vi "FWHM.vi"(3 "Peak Location":dbl, 4 "Intensity Data":dbl[](array[numeric])) -> (0 "Half Width XY Plot":cluster{dbl[], dbl[]}, 1 "Width":dbl)   [LabVIEW 2012]
panel:
  out "50% Mag - left index":dbl
  out "50% Mag - right index":dbl
  out "center -> left":dbl[](graph)
  out "center -> right":dbl[](graph)
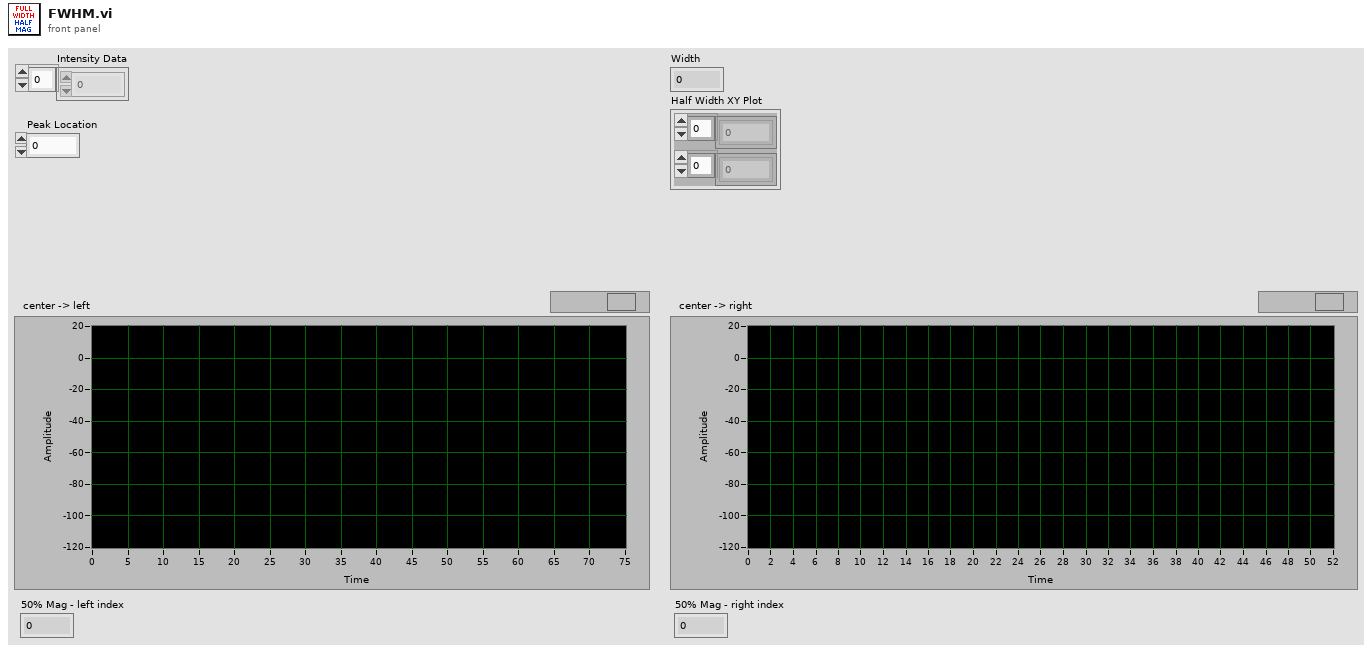
[diagram p1: front panel]
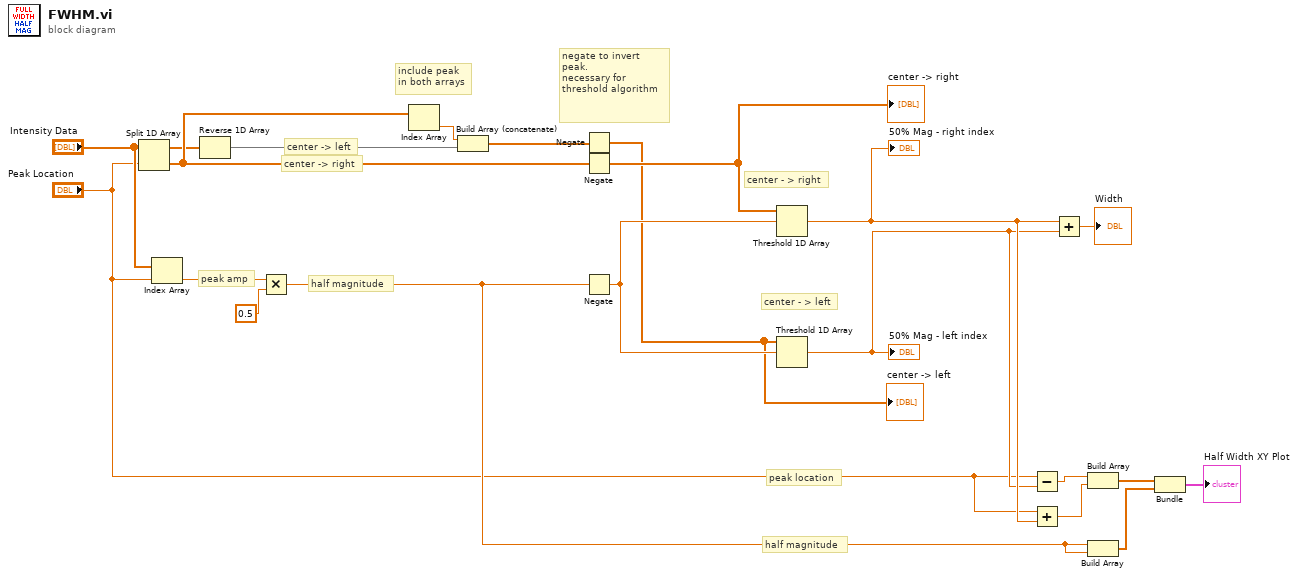
[diagram p0: block diagram]
diagram:
  # "peak amp"
  # "center -> right"
  # "center -> left"
  # "include peak\nin both arrays"
  # "negate to invert peak.\nnecessary for threshold algorithm"
  # "half magnitude"
  # "peak location"
  # "center - > left"
  # "half magnitude"
  # "center - > right"
  n1 = Split 1D Array(array="Intensity Data", index="Peak Location") -> (first subarray=w5:dbl[], second subarray=w9:dbl[])
  n2 = Index Array(array="Intensity Data", index="Peak Location") -> (element=w1:dbl)
  n3 = Reverse 1D Array(array=w5) -> (reversed array=w4:dbl[])
  n4 = Multiply(x=w1, y=0.5) -> (x*y=w13:dbl)
  n5 = Index Array(array=w9) -> (element=w8:dbl)  [unwired: 1 in]
  n6 = Build Array (concatenate)(w8, w4) -> (w7:dbl[])
  n7 = Negate(x=w7) -> (-x=w6:dbl[])
  "center -> left" <- w6
  n8 = Negate(x=w9) -> (-x=w14:dbl[])
  "center -> right" <- w14
  n9 = Negate(x=w13) -> (-x=w12:dbl)
  n10 = Threshold 1D Array(2:w12, 3:w14) -> (0:w11:dbl)  [unwired: 1 in]
  "50% Mag - right index" <- w11
  n11 = Threshold 1D Array(2:w12, 3:w6) -> (0:w10:dbl)  [unwired: 1 in]
  "50% Mag - left index" <- w10
  n12 = Subtract(x="Peak Location", y=w10) -> (x-y=w19:dbl)
  n13 = Add(x="Peak Location", y=w11) -> (x+y=w17:dbl)
  n14 = Add(x=w11, y=w10) -> (x+y=→"Width":dbl)
  n15 = Build Array(w19, w17) -> (w20:dbl[])
  n16 = Build Array(w13, w13) -> (w16:dbl[])
  n17 = Bundle(w20, w16) -> (→"Half Width XY Plot":cluster{dbl[], dbl[]})  [unwired: 1 in]
